vi "16-tcoupl_units_bis.vi"(3 "this":i32, 4 "unit in":i32, 5 "button":i32, 6 "Cluster":T1={"Auto1"=TRUE, "Auto2"=TRUE, "Rel1"=FALSE, "Rel2"=FALSE, "Filt1"=FALSE, "Filt2"=FALSE, "Rate"=enum."Slow", "Range1"=enum."10mV", "Range2"=enum."100mV", "Filt3"=FALSE, "Filt4"=FALSE, "Rel temp 1"=FALSE, "Analog1"=FALSE, "Analog2"=FALSE, "Analog temp 1"=FALSE, "Digital1"=FALSE, "Digital2"=FALSE, "Digital temp 1 "=FALSE, "Window1"=enum."None", "Window2"=enum."None", "Window temp 1"=enum."None", "RDGS1"="010", "RDGS2"="010", "RDGS temp 1"="010", "Type_type1"=TRUE, "Type_type2"=TRUE, "Type_type temp 1"=TRUE, "LSync"=FALSE, "Unit"=enum."C", "Sens"=TRUE, "Type tcoupl"=enum."J", "Junc"=TRUE, "prevState"=0, "Rel temp 2"=FALSE, "Analog temp 2"=FALSE, "Digital temp 2"=FALSE, "Type_type temp 2"=TRUE, "RDGS temp 2"="010", "Window temp 2"=enum."None", "address"="0", "digits"=0}) -> (0 "next state":i32, 1 "unit out":i32, 2 "Cluster 2":T1)   [LabVIEW 2017]
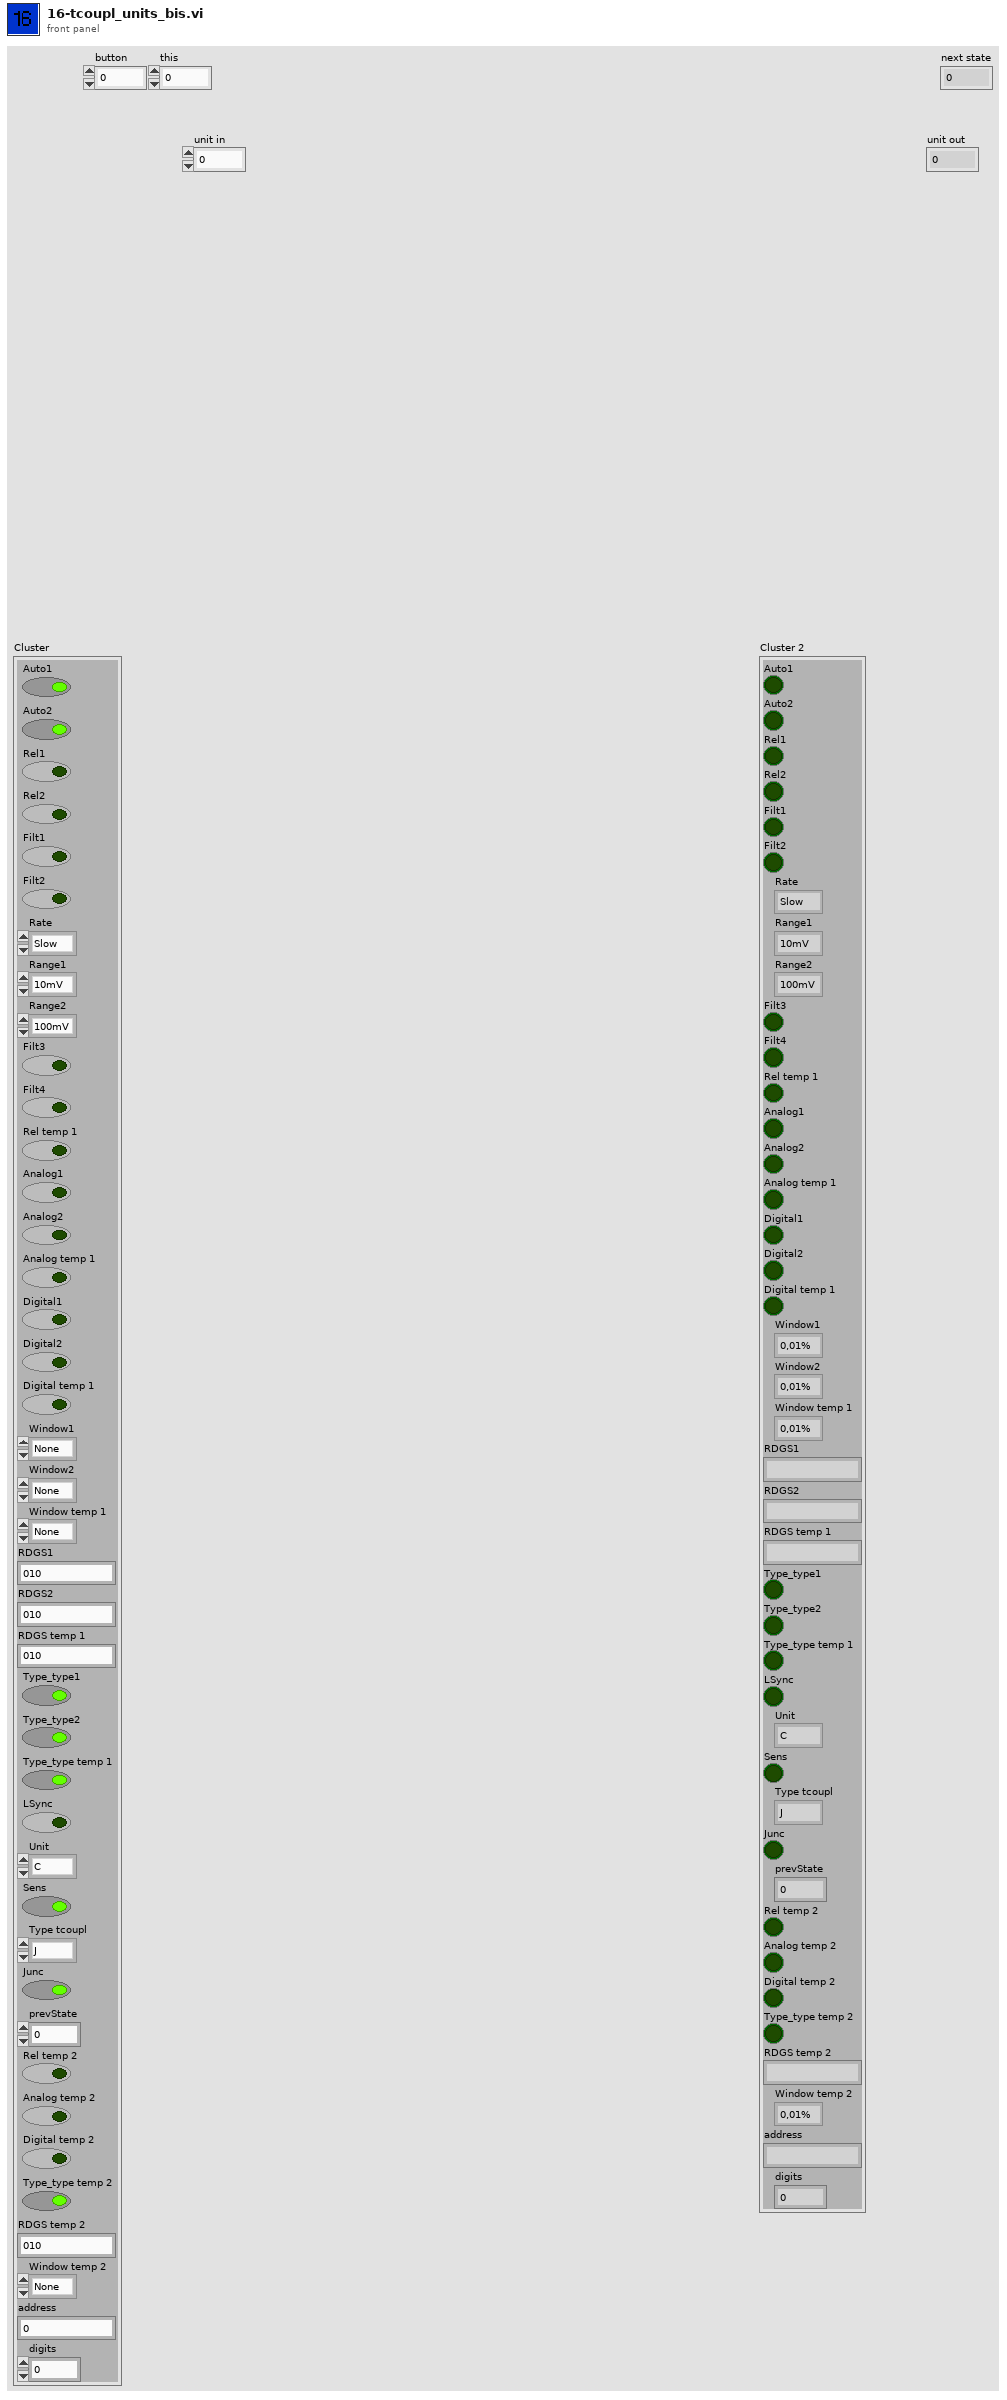
[diagram p1: front panel]
types:
  T1 = cluster{"Auto1":bool, "Auto2":bool, "Rel1":bool, "Rel2":bool, "Filt1":bool, "Filt2":bool, "Rate":enum16{"Slow", "Fast", "Med"}, "Range1":enum16{"10mV", "100mV", "1V", "10V", "100V"}, "Range2":enum16{"100mV", "1V", "10V"}, "Filt3":bool, "Filt4":bool, "Rel temp 1":bool, "Analog1":bool, "Analog2":bool, "Analog temp 1":bool, "Digital1":bool, "Digital2":bool, "Digital temp 1 ":bool, "Window1":enum16{"0,01%", "0,1%", "1%", "10%", "None"}, "Window2":enum16{"0,01%", "0,1%", "1%", "10%", "None"}, "Window temp 1":enum16{"0,01%", "0,1%", "1%", "10%", "None"}, "RDGS1":string, "RDGS2":string, "RDGS temp 1":string, "Type_type1":bool, "Type_type2":bool, "Type_type temp 1":bool, "LSync":bool, "Unit":enum16{"C", "K", "F"}, "Sens":bool, "Type tcoupl":enum16{"J", "K", "T", "E", "R", "S", "B", "N"}, "Junc":bool, "prevState":i32, "Rel temp 2":bool, "Analog temp 2":bool, "Digital temp 2":bool, "Type_type temp 2":bool, "RDGS temp 2":string, "Window temp 2":enum16{"0,01%", "0,1%", "1%", "10%", "None"}, "address":string, "digits":i32}
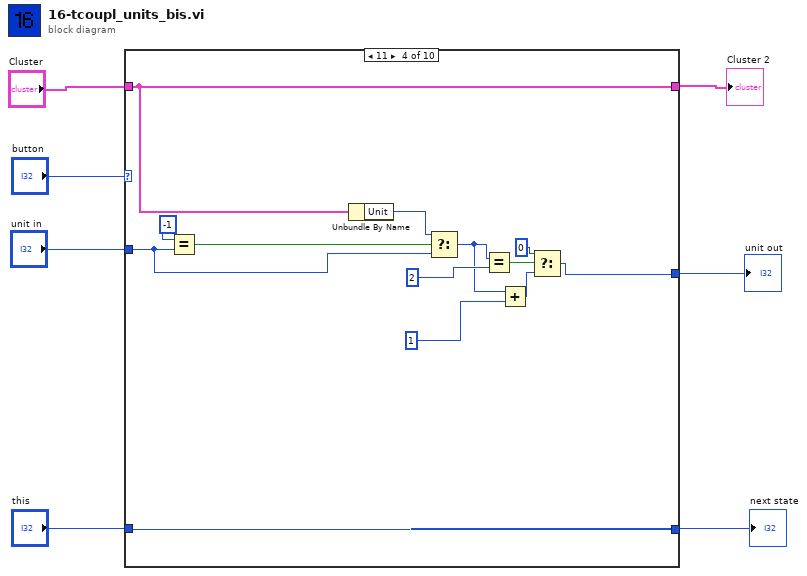
[diagram p0: block diagram]
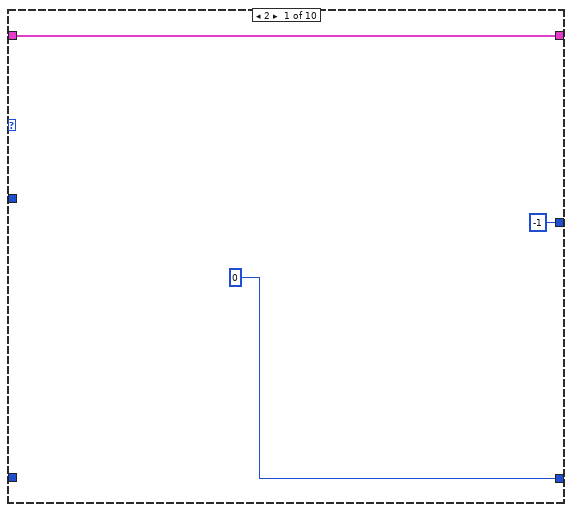
[diagram p2: hidden frame]
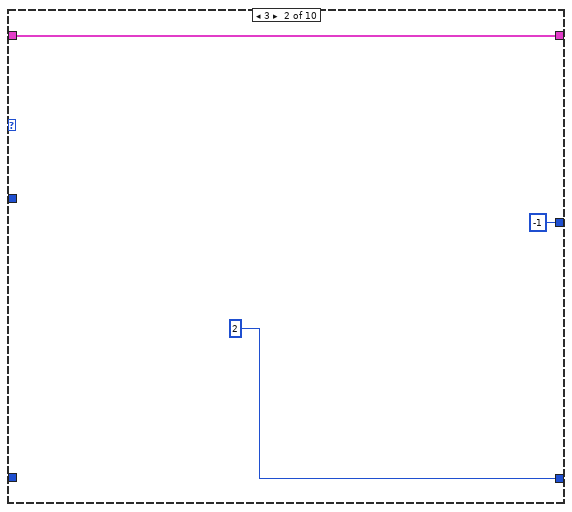
[diagram p3: hidden frame]
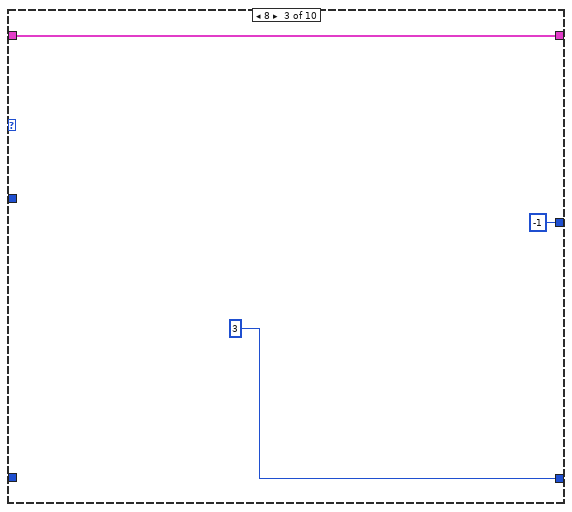
[diagram p4: hidden frame]
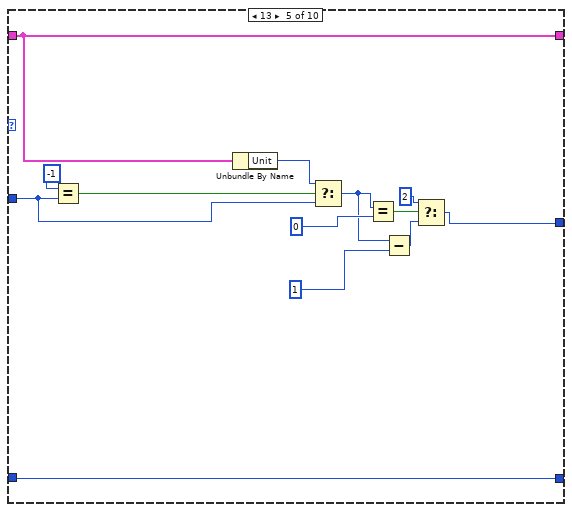
[diagram p5: hidden frame]
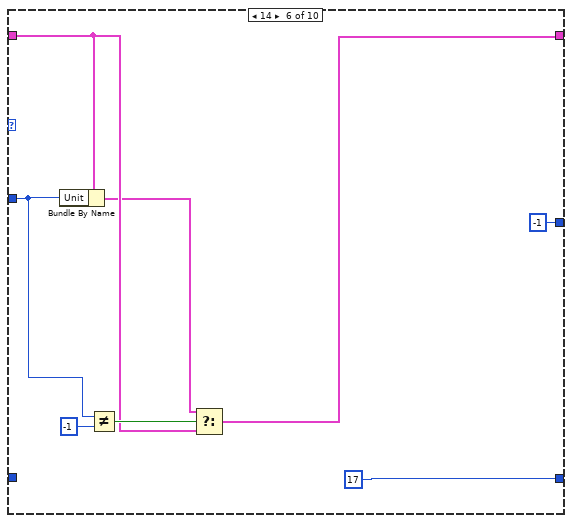
[diagram p6: hidden frame]
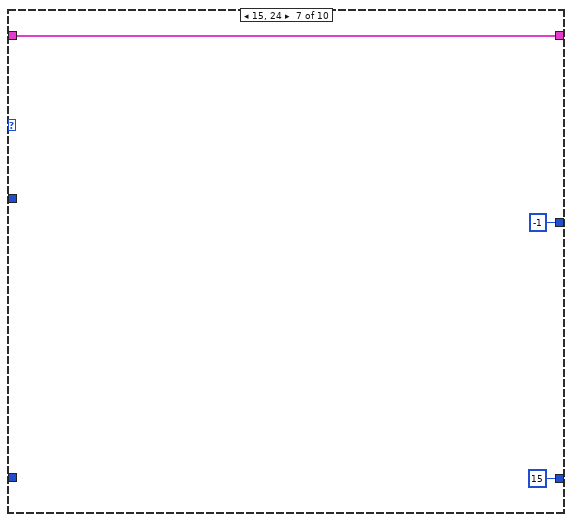
[diagram p7: hidden frame]
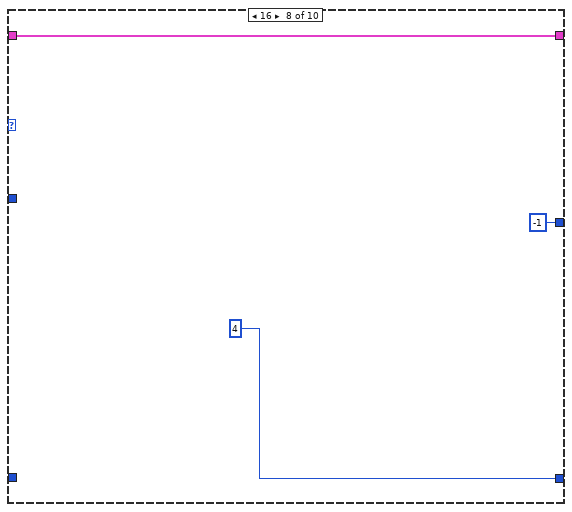
[diagram p8: hidden frame]
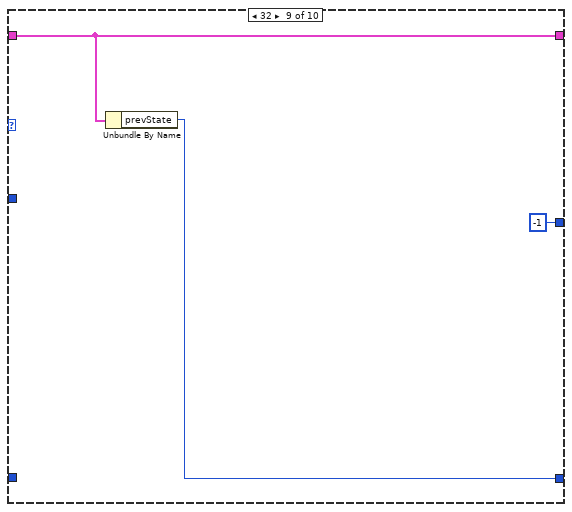
[diagram p9: hidden frame]
diagram:
  n1 = case shown="11" "button" {
    tunnel: [0 ("this") 2 3 w29 w42 17 ("this") 15 ("prevState") 4 w58 w61] -> w5
    tunnel: "this" -> [_ _ _ w29 w42 _ _ _ _ w61]
    tunnel: "Cluster" -> [w10 w12 w15 w26 w39 w47 w53 w55 w59 w62]
    tunnel: [w10 w12 w15 w26 w39 w44 w53 w55 w59 w62] -> w4
    tunnel: "unit in" -> [_ _ _ w27 w40 w46 _ _ _ w60]
    tunnel: [-1 ("window in") -1 ("window in") -1 ("window in") w24 w37 -1 ("window in") -1 ("window in") -1 ("window in") -1 ("window in") w60] -> w2
    frame 2 {
    }
    frame 3 {
    }
    frame 8 {
    }
    frame 11 {
      n2 = Equal?(x=-1, y=w27) -> (x = y?=w28:bool)
      n3 = Unbundle By Name(w26) -> ("Unit"=w18:enum16{"C", "K", "F"})
      n4 = Select(t=w18, s=w28, f=w27) -> (s? t:f=w17:i32)
      n5 = Equal?(x=w17, y=2) -> (x = y?=w22:bool)
      n6 = Add(x=w17, y=1) -> (x+y=w23:i32)
      n7 = Select(t=0, s=w22, f=w23) -> (s? t:f=w24:i32)
    }
    frame 13 {
      n8 = Equal?(x=-1, y=w40) -> (x = y?=w41:bool)
      n9 = Unbundle By Name(w39) -> ("Unit"=w31:enum16{"C", "K", "F"})
      n10 = Select(t=w31, s=w41, f=w40) -> (s? t:f=w30:i32)
      n11 = Equal?(x=w30, y=0) -> (x = y?=w35:bool)
      n12 = Subtract(x=w30, y=1) -> (x-y=w36:i32)
      n13 = Select(t=2, s=w35, f=w36) -> (s? t:f=w37:i32)
    }
    frame 14 {
      n14 = Bundle By Name(cluster=w47, "Unit"=w46) -> (w45:T1)
      n15 = Not Equal?(x=w46, y=-1) -> (x != y?=w48:bool)
      n16 = Select(t=w45, s=w48, f=w47) -> (s? t:f=w44:T1)
    }
    frame 15, 24 {
    }
    frame 16 {
    }
    frame 32 {
      n17 = Unbundle By Name(w59) -> ("prevState"=w58:i32)
    }
    frame Default {
    }
  }
  "next state" <- w5
  "unit out" <- w2
  "Cluster 2" <- w4
